vi "Query Mouse Position.vi"(8 "error in (no error)":errorcluster, 10 "key mode":enum16{"RELATIVE", "ABSOLUTE"}(ring)=enum."ABSOLUTE", 11 "device ID 2":refnum<k1>) -> (0 "error out":errorcluster, 1 "button info":T1, 2 "axis info":T2, 3 "device ID":refnum<k1>)   [LabVIEW 2015]
uses:
  <resource>/lvinput.dll
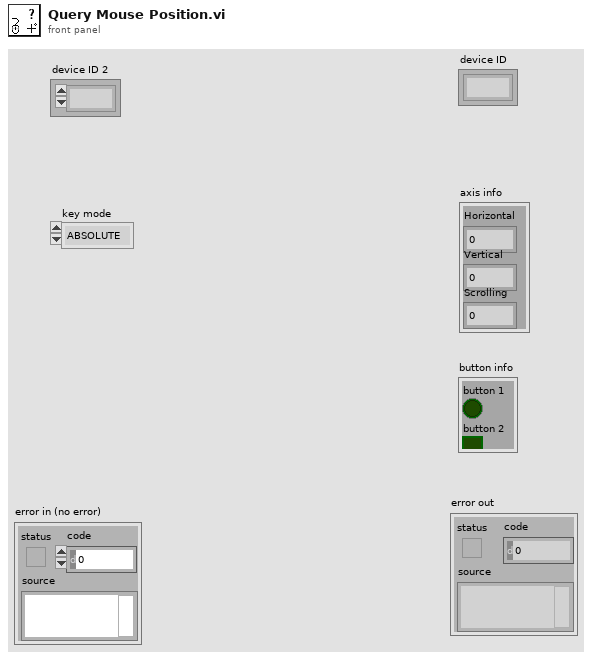
[diagram p1: front panel]
types:
  T1 = cluster{"button 1":bool, "button 2":bool, "button 3":bool, "button 4":bool}
  T2 = cluster{"Horizontal":i32, "Vertical":i32, "Scrolling":i32}
  T3 = cluster{"[0]":bool, "[1]":bool, "[2]":bool, "[3]":bool}
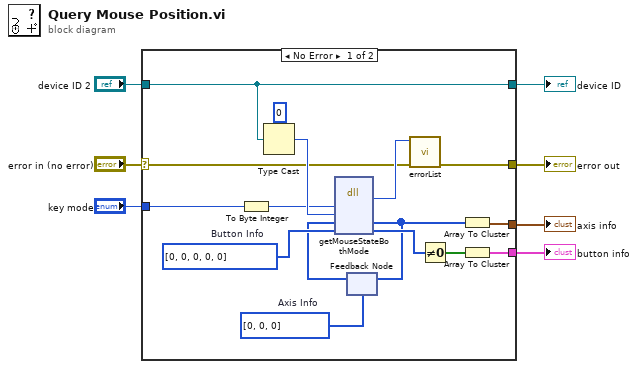
[diagram p0: block diagram]
diagram:
  n1 = case shown="No Error" "error in (no error)" {
    selector: "error in (no error)" -> [w11 w24]
    tunnel: [w14 w24] -> w7
    tunnel: [w17 cluster{i32, i32, i32} {0, 0, 0}] -> w5
    tunnel: [w15 cluster{bool, bool, bool, bool} {FALSE, FALSE, FALSE, FALSE}] -> w3
    tunnel: "device ID 2" -> [w12 w25]
    tunnel: [w12 w25] -> w2
    tunnel: "key mode" -> [w13 _]
    frame No Error {
      w8 = i32[] [0, 0, 0]  # Axis Info
      w20 = i8[] [0, 0, 0, 0, 0]  # Button Info
      n2 = To Byte Integer(number=w13) -> (8bit integer=w18:i8)
      n3 = Type Cast(type=0, x=w12) -> (*(type *) &x=w21:i32)
      n4 = feedback #1(w8) -> (w9:i32[])
      n5 = dll-call lib="D:/LabVIEW 2015/resource/lvinput.*" fn="getMouseStateBothMode"(w18, w21, w9, w20) -> (w23:i32, w10:i32[], w19:i8[])  [unwired: 5 in, 2 out]
      n6 = feedback-in #1(w10) -> ()
      n7 = call <vilib>:"errorList.vi"("error in (no error)"=w11, "error code"=w23) -> ("error out"=w14:errorcluster)  [unwired: 9 in]
      n8 = Not Equal To 0?(x=w19) -> (x != 0?=w16:bool[])
      n9 = Array To Cluster(array=w10) -> (cluster=w17:cluster{"[0]":i32, "[1]":i32, "[2]":i32})
      n10 = Array To Cluster(array=w16) -> (cluster=w15:T3)
    }
    frame Error {
    }
  }
  "error out" <- w7
  "axis info" <- w5
  "button info" <- w3
  "device ID" <- w2
